vi "PC-Based UDP Sending Sensors.vi"() -> ()   [LabVIEW 2009]
uses:
  UDP3-GPS, INS/UDP 3.ctl
  UDP3-GPS, INS/UDP3GLOB.vi
panel:
  out "UDP Heartbeat":bool
  in  "GPS Main Loop Timer (ms)":u32=40
  out "UDP 3":T1
  out "GPS Heartbeat":bool
  in  "stop":bool
  in  "VISA resource name 2":refnum<visa-resource-name>="COM5"
  in  "VISA resource name":refnum<visa-resource-name>="COM6"
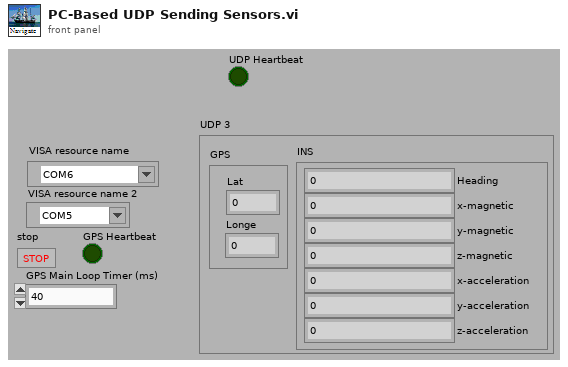
[diagram p1: front panel]
types:
  T1 = typedef "UDP 3.ctl" = cluster{"GPS":cluster{"Lat":dbl, "Longe":dbl}, "INS":cluster{"Heading":dbl, "x-magnetic":dbl, "y-magnetic":dbl, "z-magnetic":dbl, "x-acceleration":dbl, "y-acceleration":dbl, "z-acceleration":dbl}}
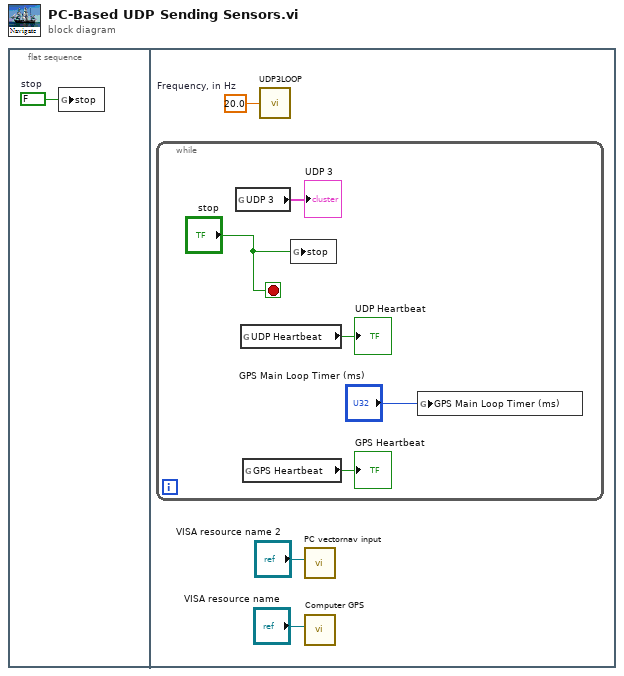
[diagram p0: block diagram]
diagram:
  n1 = flat-sequence {
    frame #0 {
      w1 = FALSE  # stop
      n2 = global write "UDP3GLOB.vi" "stop"(w1) -> ()
    }
    frame #1 {
      w4 = 20.0  # Frequency, in Hz
      n3 = while {
        stop <- "stop" stop-if-true
        n4 = global read "UDP3GLOB.vi" "UDP 3"() -> (→"UDP 3":T1)
        n5 = global read "UDP3GLOB.vi" "UDP Heartbeat"() -> (→"UDP Heartbeat":bool)
        n6 = global read "UDP3GLOB.vi" "GPS Heartbeat"() -> (→"GPS Heartbeat":bool)
        n7 = global write "UDP3GLOB.vi" "stop"("stop") -> ()
        n8 = global write "UDP3GLOB.vi" "GPS Main Loop Timer (ms)"("GPS Main Loop Timer (ms)") -> ()
      }
      n9 = call "UDP3LOOP.vi"("Frequency, in Hz"=w4) -> ()
      n10 = call "PC vectornav input.vi"("VISA resource name"="VISA resource name 2") -> ()  [unwired: 11 in]
      n11 = call "Computer GPS.vi"("VISA resource name"="VISA resource name") -> ()  [unwired: 11 in]
    }
  }
